vi "test Copy.vi"(8 "error in (no error)":errorcluster, 11 "TestCase in":refnum<class "Buffers Tests.lvclass">) -> (0 "error out":errorcluster, 3 "TestCase out":refnum<class "Buffers Tests.lvclass">)   [LabVIEW 2017, in "Buffers Tests.lvclass"]
uses:
  Buffers Tests.lvclass
  Buffers Tests.lvclass/Buffers Tests.ctl
  Classes/Buffers/Buffers.lvclass/Buffers.ctl
  <vilib>/NI/Memory Manager/Classes/Pointer/Pointer.lvclass/Pointer.ctl
  <vilib>/NI/Memory Manager/Classes/Pointer/Get Size.vi
  <vilib>/NI/Memory Manager/Classes/Pointer/Copy All.vi
  <vilib>/NI/Memory Manager/Classes/Pointer/Clear.vi
  <vilib>/NI/Memory Manager/Classes/Pointer/Copy.vi
  <vilib>/NI/Memory Manager/Classes/Pointer/Check Null Pointer.vi
  <vilib>/NI/Memory Manager/Classes/Pointer/Clear (No Check).vi
  <vilib>/NI/Memory Manager/Classes/Pointer/Check Length.vi
  <vilib>/NI/Memory Manager/Classes/Pointer/Copy (No Check).vi
  <vilib>/NI/Memory Manager/Classes/Pointer/Check Bounds (Pointer).vi
  <vilib>/NI/Memory Manager/Classes/Pointer/Errors.vi
  <vilib>/NI/Memory Manager/Classes/Pointer/Null Pointer.vi
  <vilib>/NI/Memory Manager/Classes/Pointer/Is Null.vi
  <vilib>/NI/Memory Manager/Classes/Pointer/Get Address.vi
  <vilib>/NI/Memory Manager/Classes/Pointer/Out of Bounds.vi
  <vilib>/NI/Memory Manager/Classes/Pointer/Create Error.vi
  <vilib>/NI/Memory Manager/Classes/Pointer/Write Pointer Size to Error.vi
  <vilib>/NI/Memory Manager/Constants/Constants.vi
  <vilib>/NI/Memory Manager/Constants/Library Name.vi
  <vilib>/NI/Memory Manager/Classes/Pointer/Pointer Error Info.vi
  <vilib>/NI/Memory Manager/Constants/Pointer Class Name.vi
  Classes/Buffer/Buffer.lvclass
  C:/Program Files (x86)/National Instruments/LabVIEW 2017/vi.lib/NI/Memory Manager/Classes/Pointer/Pointer.lvclass
  Classes/Buffer/Write Buffer 1D U8.vi
  <vilib>/NI/Memory Manager/VIs/New Error Cluster.vi
  <vilib>/NI/Memory Manager/VIs/New Error Cluster (512B).vi
  <vilib>/NI/Memory Manager/VIs/Set Error Status.vi
  <vilib>/NI/Memory Manager/VIs/Set Error Code.vi
  <vilib>/NI/Memory Manager/VIs/Set Error Source.vi
  <vilib>/NI/Memory Manager/VIs/Write String to Source.vi
  <vilib>/NI/Memory Manager/VIs/Write Numeric to Source.vi
  <vilib>/NI/Memory Manager/VIs/Write Numeric Scalar to Source (Base10 U64).vi
  Classes/Buffer/Read Buffer 1D U8.vi
  <vilib>/addons/_JKI Toolkits/VI Tester/TestCase.llb/TestCase.lvclass
  Classes/Buffers/Buffers.lvclass
  C:/Program Files (x86)/National Instruments/LabVIEW 2017/vi.lib/addons/_JKI Toolkits/VI Tester/TestCase.llb/TestCase.lvclass
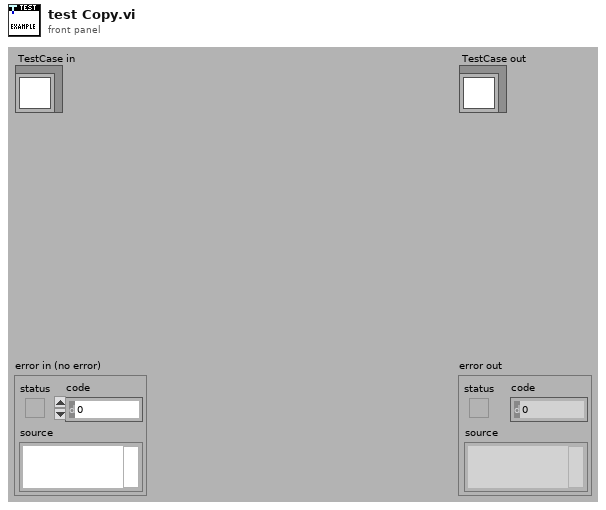
[diagram p1: front panel]
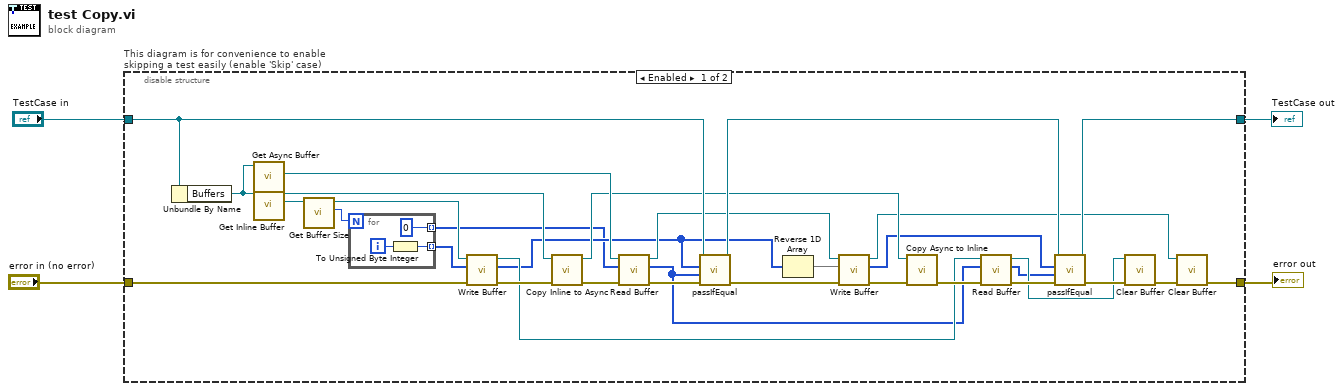
[diagram p0: block diagram]
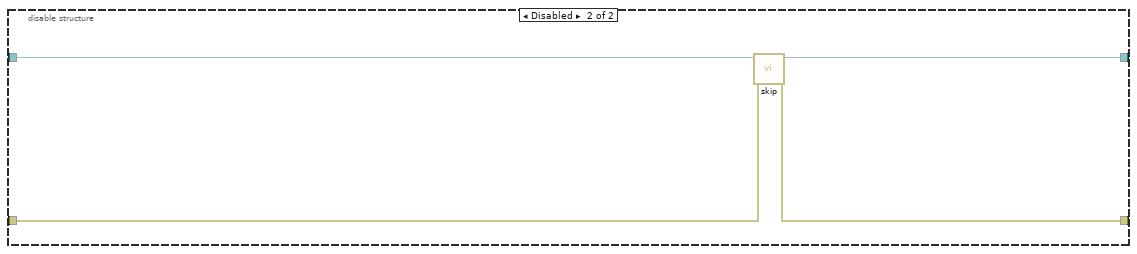
[diagram p2: hidden frame]
diagram:
  n1 = disable-structure "This diagram is for convenience to enable skipping a test easily (enable 'Skip' case)" shown="Enabled" {
    disable-tunnel: "TestCase in" -> [w17 w43]
    disable-tunnel: [w36 w41] -> w1
    disable-tunnel: [w5 w42] -> w3
    disable-tunnel: "error in (no error)" -> [w35 w40]
    frame Enabled {
      n2 = Unbundle By Name(w17) -> ("Buffers"=w34:refnum<class "Buffers.lvclass">)
      n3 = call "Get Async Buffer.vi"("Buffers in"=w34) -> ("Async Buffer"=w26:refnum<class "Buffer.lvclass">)  [unwired: 9 in, 1 out]
      n4 = call "Get Inline Buffer.vi"("Buffers in"=w34) -> ("Inline Buffer"=w32:refnum<class "Buffer.lvclass">, "Buffers out"=w33:refnum<class "Buffers.lvclass">)  [unwired: 9 in]
      n5 = call "Get Buffer Size.vi"("Buffer in"=w32) -> ("buffer size"=w30:u64, "Buffer out"=w31:refnum<class "Buffer.lvclass">)  [unwired: 9 in]
      n6 = for {
        N: w30 -> [_]
        tunnel: [w38] -> w29 mode=indexing
        tunnel: [u8 0] -> w12 mode=indexing
        i -> [w39]
        n7 = To Unsigned Byte Integer(number=w39) -> (unsigned 8bit integer=w38:u8)
      }
      n8 = call-poly "Write Buffer.vi"("error in (no error)"=w35, "src array in"=w29, "Buffer in"=w31) -> ("error out"=w28:errorcluster, "src array out"=w13:u8[], "Buffer out"=w20:refnum<class "Buffer.lvclass">)  [unwired: 5 in, 1 out]
      n9 = call "Copy Inline to Async.vi"("error in (no error)"=w28, "Buffers in"=w33) -> ("error out"=w27:errorcluster, "Buffers out"=w14:refnum<class "Buffers.lvclass">)  [unwired: 8 in]
      n10 = call-poly "Read Buffer.vi"("error in (no error)"=w27, "dst array in"=w12, "Buffer in"=w26) -> ("error out"=w25:errorcluster, "dst array out"=w19:u8[], "Buffer out"=w15:refnum<class "Buffer.lvclass">)  [unwired: 5 in, 1 out]
      n11 = call-dynamic "passIfEqual.vi"("error in (no error)"=w25, "y"=w19, "x"=w13, "TestCase in"=w17) -> ("error out"=w24:errorcluster, "TestCase out"=w16:refnum<class "Buffers Tests.lvclass">)  [unwired: 6 in]
      n12 = Reverse 1D Array(array=w13) -> (reversed array=w23:u8[])
      n13 = call-poly "Write Buffer.vi"("error in (no error)"=w24, "src array in"=w23, "Buffer in"=w15) -> ("error out"=w22:errorcluster, "src array out"=w11:u8[], "Buffer out"=w6:refnum<class "Buffer.lvclass">)  [unwired: 5 in, 1 out]
      n14 = call "Copy Async to Inline.vi"("error in (no error)"=w22, "Buffers in"=w14) -> ("error out"=w21:errorcluster)  [unwired: 8 in, 1 out]
      n15 = call-poly "Read Buffer.vi"("error in (no error)"=w21, "dst array in"=w19, "Buffer in"=w20) -> ("error out"=w18:errorcluster, "dst array out"=w7:u8[], "Buffer out"=w8:refnum<class "Buffer.lvclass">)  [unwired: 5 in, 1 out]
      n16 = call-dynamic "passIfEqual.vi"("error in (no error)"=w18, "y"=w7, "x"=w11, "TestCase in"=w16) -> ("error out"=w10:errorcluster, "TestCase out"=w36:refnum<class "Buffers Tests.lvclass">)  [unwired: 6 in]
      n17 = call "Clear Buffer.vi"("error in (no error)"=w10, "Buffer in"=w8) -> ("error out"=w9:errorcluster)  [unwired: 8 in, 1 out]
      n18 = call "Clear Buffer.vi"("error in (no error)"=w9, "Buffer in"=w6) -> ("error out"=w5:errorcluster)  [unwired: 8 in, 1 out]
    }
    frame Disabled {
      # "skip test result while test is under development"
      n19 = call <vilib>:"skip.vi"("error in (no error)"=w40, "TestCase in"=w43) -> ("error out"=w42:errorcluster, "TestCase out"=w41:refnum<class "Buffers Tests.lvclass">)  [unwired: 8 in]
    }
  }
  "error out" <- w3
  "TestCase out" <- w1
